vi "状态告警区转CDAB.vi"(11 "状态告警区":T1) -> (3 "输出数组":u16[](array[numeric]))   [LabVIEW 2016]
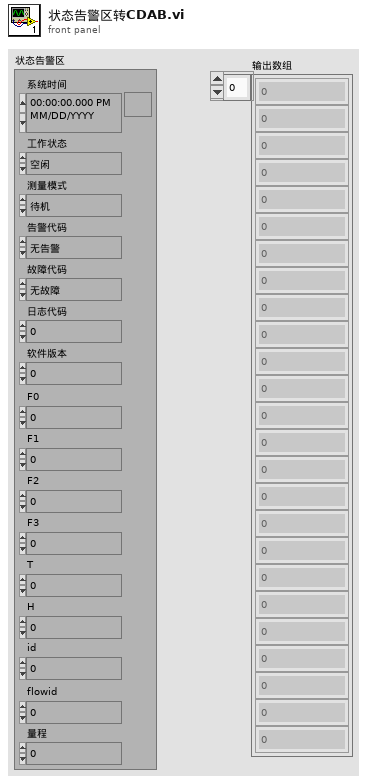
[diagram p1: front panel]
types:
  T1 = cluster{"系统时间":timestamp, "工作状态":enum16{"空闲", "水样测试", "标样核查", "零点核查", "跨度核查", "空白测试", "平行样测试", "加标回收", "空白校准", "标样校准", "初始化（清洗）"}, "测量模式":enum16{"待机", "连续模式", "周期模式", "定点模式", "受控模式", "手动模式"}, "告警代码":enum16{"无告警", "缺试剂告警", "缺水样告警", "缺蒸馏水告警", "缺标液告警", "仪表漏液告警", "标定异常告警", "超量程告警", "加热异常", "低试剂预警", "超上限告警", "超下限告警", "仪表内部其他异常", "滴定异常告警", "电极异常告警", "量程切换告警", "参数设置告警", "PH电极电位异常", "电导率电极异常", "浊度光度异常", "溶解氧电极异常", "溶解氧光强异常", "温度异常告警", "PH异常告警", "溶解氧异常告警", "电导率异常告警", "浊度异常告警", "叶绿素异常告警", "藻密度异常告警", "蓝绿藻异常告警", "ORP异常告警", "氨氮异常告警", "清洁刷异常告警", "SD卡异常告警", "蓝牙异常告警", "Wifi异常告警", "流程异常告警"}, "故障代码":enum16{"无故障", "电机故障", "温度故障", "通讯故障", "滴定故障"}, "日志代码":u16, "软件版本":u16, "F0":sgl, "F1":sgl, "F2":sgl, "F3":sgl, "T":sgl, "H":sgl, "id":u16, "flowid":u16, "量程":u16}
  T2 = enum16{"空闲", "水样测试", "标样核查", "零点核查", "跨度核查", "空白测试", "平行样测试", "加标回收", "空白校准", "标样校准", "初始化（清洗）"}
  T3 = enum16{"待机", "连续模式", "周期模式", "定点模式", "受控模式", "手动模式"}
  T4 = enum16{"无告警", "缺试剂告警", "缺水样告警", "缺蒸馏水告警", "缺标液告警", "仪表漏液告警", "标定异常告警", "超量程告警", "加热异常", "低试剂预警", "超上限告警", "超下限告警", "仪表内部其他异常", "滴定异常告警", "电极异常告警", "量程切换告警", "参数设置告警", "PH电极电位异常", "电导率电极异常", "浊度光度异常", "溶解氧电极异常", "溶解氧光强异常", "温度异常告警", "PH异常告警", "溶解氧异常告警", "电导率异常告警", "浊度异常告警", "叶绿素异常告警", "藻密度异常告警", "蓝绿藻异常告警", "ORP异常告警", "氨氮异常告警", "清洁刷异常告警", "SD卡异常告警", "蓝牙异常告警", "Wifi异常告警", "流程异常告警"}
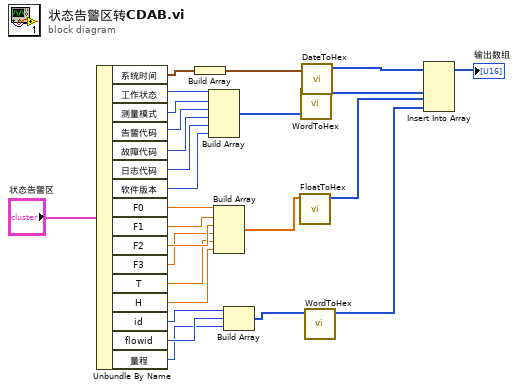
[diagram p0: block diagram]
diagram:
  n1 = Unbundle By Name("状态告警区") -> ("系统时间"=w25:timestamp, "工作状态"=w22:T2, "测量模式"=w19:T3, "告警代码"=w18:T4, "故障代码"=w17:enum16{"无故障", "电机故障", "温度故障", "通讯故障", "滴定故障"}, "日志代码"=w16:u16, "软件版本"=w15:u16, "F0"=w14:sgl, "F1"=w12:sgl, "F2"=w11:sgl, "F3"=w10:sgl, "T"=w9:sgl, "H"=w8:sgl, "id"=w6:u16, "flowid"=w5:u16, "量程"=w4:u16)
  n2 = Build Array(w25) -> (w24:timestamp[])
  n3 = Build Array(w22, w19, w18, w17, w16, w15) -> (w21:u16[])
  n4 = Build Array(w14, w12, w11, w10, w9, w8) -> (w13:sgl[])
  n5 = Build Array(w6, w5, w4) -> (w3:u16[])
  n6 = call "FloatToHex.vi"("浮点数"=w13) -> ("DCBA整形输出"=w7:u16[])  [unwired: 10 in]
  n7 = call "WordToHex.vi"("WORD"=w21) -> ("数组"=w20:u16[])  [unwired: 10 in]
  n8 = call "DateToHex.vi"("DATE"=w24) -> ("数组"=w23:u16[])  [unwired: 10 in]
  n9 = call "WordToHex.vi"("WORD"=w3) -> ("数组"=w2:u16[])  [unwired: 10 in]
  n10 = Insert Into Array(array=w23, new element #1=w20, new element #2=w7, new element #3=w2) -> (→"输出数组":u16[])  [unwired: 1 in]
